vi "Save to file.vi"(10 "String":string, 11 "Control panel":T1) -> ()   [LabVIEW 2020]
uses:
  <vilib>/Utility/file.llb/Write Delimited Spreadsheet (string).vi
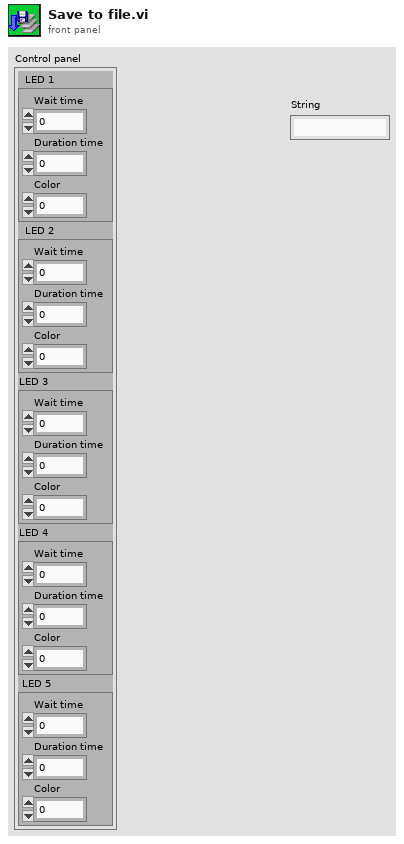
[diagram p1: front panel]
types:
  T1 = cluster{"  LED 1":cluster{"Wait time":dbl, "Duration time":dbl, "Color":u32}, "  LED 2":cluster{"Wait time":dbl, "Duration time":dbl, "Color":u32}, "LED 3":cluster{"Wait time":dbl, "Duration time":dbl, "Color":u32}, "LED 4":cluster{"Wait time":dbl, "Duration time":dbl, "Color":u32}, " LED 5":cluster{"Wait time":dbl, "Duration time":dbl, "Color":u32}}
  T2 = enum16{"open", "replace", "create", "open or create", "replace or create", "replace or create with confirmation"}
  T3 = cluster{"Wait time":dbl, "Duration time":dbl, "Color":u32}
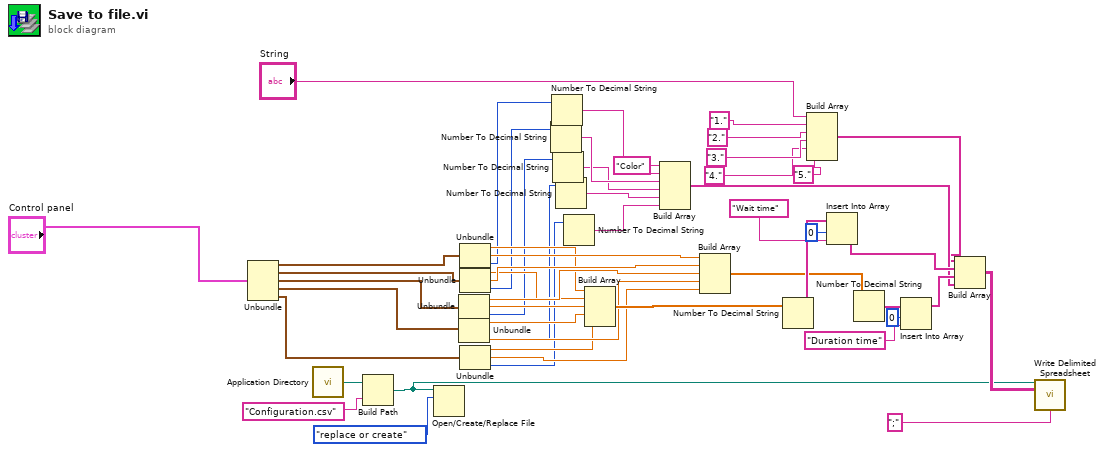
[diagram p0: block diagram]
diagram:
  n1 = Unbundle("Control panel") -> ("LED 1"=w29:T3, "LED 2"=w30:T3, "LED 3"=w31:T3, "LED 4"=w32:T3, "LED 5"=w33:T3)
  n2 = call <vilib>:"Application Directory.vi"() -> ("Application Directory"=w26:path)
  n3 = Build Path(base path=w26, name or relative path="Configuration.csv") -> (appended path=w39:path)
  n4 = Open/Create/Replace File(file path (use dialog)=w39, operation (0:open)=T2."replace or create") -> ()  [unwired: 4 in, 3 out]
  n5 = Unbundle(w31) -> ("Wait time"=w36:dbl, "Duration time"=w43:dbl, "Color"=w17:u32)
  n6 = Unbundle(w32) -> ("Wait time"=w37:dbl, "Duration time"=w44:dbl, "Color"=w16:u32)
  n7 = Unbundle(w29) -> ("Wait time"=w34:dbl, "Duration time"=w41:dbl, "Color"=w19:u32)
  n8 = Unbundle(w30) -> ("Wait time"=w35:dbl, "Duration time"=w42:dbl, "Color"=w18:u32)
  n9 = Unbundle(w33) -> ("Wait time"=w38:dbl, "Duration time"=w45:dbl, "Color"=w15:u32)
  n10 = Number To Decimal String(number=w18) -> (decimal integer string=w13:string)  [unwired: 1 in]
  n11 = Number To Decimal String(number=w19) -> (decimal integer string=w14:string)  [unwired: 1 in]
  n12 = Number To Decimal String(number=w17) -> (decimal integer string=w12:string)  [unwired: 1 in]
  n13 = Number To Decimal String(number=w16) -> (decimal integer string=w11:string)  [unwired: 1 in]
  n14 = Number To Decimal String(number=w15) -> (decimal integer string=w10:string)  [unwired: 1 in]
  n15 = Build Array(w34, w35, w36, w37, w38) -> (w47:dbl[])
  n16 = Build Array("Color" ("element"), w14, w13, w12, w11, w10) -> (w8:string[])
  n17 = Build Array(w41, w42, w43, w44, w45) -> (w48:dbl[])
  n18 = Number To Decimal String(number=w47) -> (decimal integer string=w49:string[])  [unwired: 1 in]
  n19 = Build Array("String", "1.", "2.", "3.", "4.", "5.") -> (w6:string[])
  n20 = Insert Into Array(array=w49, index=0, new element="Wait time" ("new element/subarray")) -> (w50:string[])
  n21 = Number To Decimal String(number=w48) -> (decimal integer string=w24:string[])  [unwired: 1 in]
  n22 = Insert Into Array(array=w24, index=0, new element="Duration time" ("new element/subarray")) -> (w23:string[])
  n23 = Build Array(w6, w50, w23, w8) -> (w46:string[][])
  n24 = call-poly <vilib>:"Write Delimited Spreadsheet.vi"("file path (dialog if empty)"=w39, "2D data"=w46, "delimiter (\\t)"=";" ("delimiter (\\t)")) -> ()  [unwired: 11 in, 2 out]
